vi "_Lookup Double Channel.vi"(8 "error in (no error)":errorcluster, 10 "Channel Name":string, 11 "Loop Data in":T1) -> (0 "error out":errorcluster, 2 "Channel":refnum<class "Channel.lvclass">, 3 "Loop Data":T1)   [LabVIEW 2020, in "Vecto.lvlib" / "ChannelService.lvclass"]
uses:
  ChannelService.lvclass
  ChannelService.lvclass/ChannelService.ctl
  Group/Group.lvclass
  Loop Data.ctl
  Channel/Channel.lvclass
  GroupAbstract/GroupAbstract.lvclass
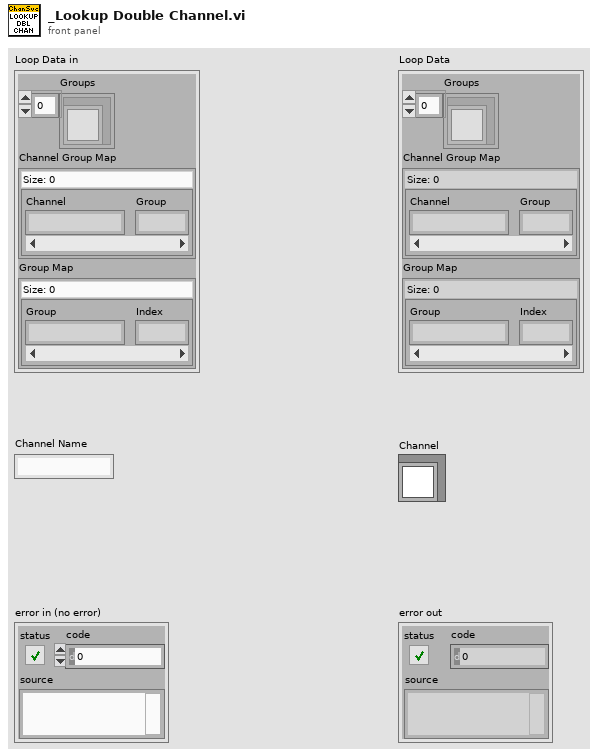
[diagram p1: front panel]
types:
  T1 = typedef "Vecto.lvlib/ChannelService.lvclass/Loop Data.ctl" = cluster{"Groups":refnum<class "GroupAbstract.lvclass">[], "Channel Group Map":map{string, i32}, "Group Map":map{string, i32}}
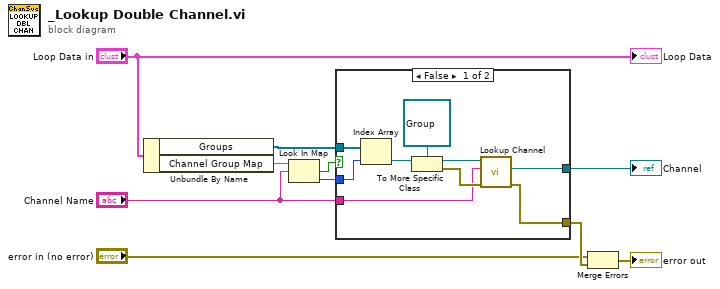
[diagram p0: block diagram]
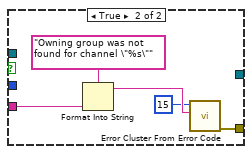
[diagram p2: hidden frame]
diagram:
  n1 = Unbundle By Name("Loop Data in") -> ("Groups"=w7:refnum<class "GroupAbstract.lvclass">[], "Channel Group Map"=w10:map{string, i32})
  n2 = Look In Map(map=w10, key="Channel Name") -> (key not found?=w9:bool, value=w8:i32)  [unwired: 1 in]
  n3 = case shown="False" w9 {
    tunnel: w8 -> [w17 _]
    tunnel: w7 -> [w18 _]
    tunnel: "Channel Name" -> [w15 w24]
    tunnel: [w14 _] -> w4
    tunnel: [w13 w20] -> w3
    frame False {
      n4 = Index Array(array=w18, index=w17) -> (element=w16:refnum<class "GroupAbstract.lvclass">)
      n5 = To More Specific Class(target class=refnum<class "Group.lvclass"> refnum ("Vecto.lvlib:Group.lvclass"), reference=w16) -> (specific class reference=w12:refnum<class "Group.lvclass">, error out=w19:errorcluster)  [unwired: 1 in]
      n6 = call "Lookup Channel.vi"("error in (no error)"=w19, "Channel Name"=w15, "Group in"=w12) -> ("error out"=w13:errorcluster, "Channel"=w14:refnum<class "Channel.lvclass">)  [unwired: 6 in, 1 out]
    }
    frame True {
      n7 = Format Into String(format string="Owning group was not found for channel \"%s\"", w24) -> (resulting string=w22:string)  [unwired: 2 in, 1 out]
      n8 = call <vilib>:"Error Cluster From Error Code.vi"("error message (\"\")"=w22, "error code (0)"=15) -> ("error out"=w20:errorcluster)  [unwired: 7 in]
    }
  }
  "Channel" <- w4
  n9 = Merge Errors("error in (no error)", w3) -> (→"error out":errorcluster)
  "Loop Data" <- "Loop Data in"
